vi "Function data mismatch error1.vi"(8 "error in (no error)":errorcluster) -> (0 "error out":errorcluster)   [LabVIEW 2019, in "NI_modbus_upd.lvlib"]
doc: "Throws error when called. This error should be used to indicate that the returned data (ie for write functions) does not match the data sent."
uses:
  NI_modbus_upd.lvlib
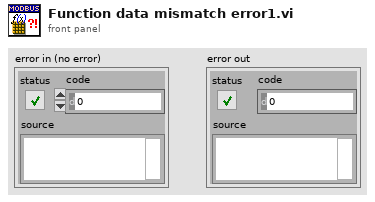
[diagram p1: front panel]
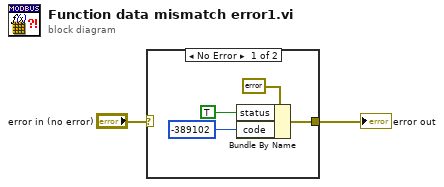
[diagram p0: block diagram]
diagram:
  n1 = case shown="No Error" "error in (no error)" {
    selector: "error in (no error)" -> [_ w7]
    tunnel: [w3 w7] -> w1
    frame No Error {
      n2 = Bundle By Name(cluster=errorcluster {"status"=FALSE, "code"=0, "source"=""} ("error constant"), "status"=TRUE, "code"=-389102) -> (w3:errorcluster)
    }
    frame Error {
    }
  }
  "error out" <- w1
